vi "Process Init.vi"(0 "Process In":refnum<class "Process.lvclass">, 7 "Process Name":string, 11 "Error In":errorcluster) -> (4 "Process Out":refnum<class "Process.lvclass">, 15 "Error Out":errorcluster)   [LabVIEW 2023, in "Process.lvclass"]
doc: "Initializes new process by naming and starting it."
uses:
  Process.lvclass
  Process.lvclass/Process.ctl
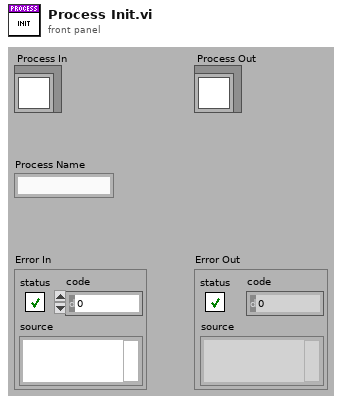
[diagram p1: front panel]
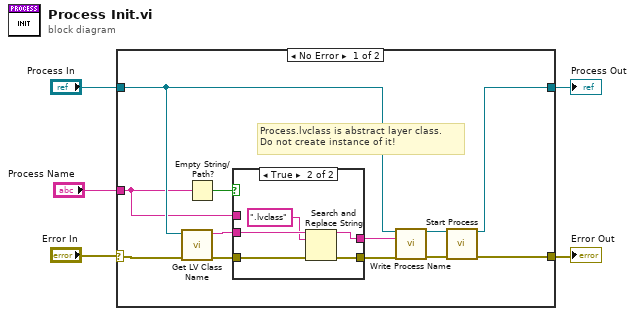
[diagram p0: block diagram]
diagram:
  n1 = case shown="No Error" "Error In" {
    selector: "Error In" -> [w10 w25]
    tunnel: "Process In" -> [w13 w26]
    tunnel: [w16 w26] -> w4
    tunnel: [w17 w25] -> w2
    tunnel: "Process Name" -> [w6 _]
    frame No Error {
      # "Process.lvclass is abstract layer class. \nDo not create instance of it!"
      n2 = call <vilib>:"Get LV Class Name.vi"("error in (no error)"=w10, "object"=w13) -> ("error out"=w9:errorcluster, "class name"=w11:string)  [unwired: 8 in]
      n3 = Empty String/Path?(string/path=w6) -> (empty?=w7:bool)
      n4 = case shown="True" w7 {
        tunnel: w6 -> [w19 _]
        tunnel: [w19 w22] -> w12
        tunnel: w11 -> [_ w24]
        tunnel: w9 -> [w18 w21]
        tunnel: [w18 w20] -> w8
        frame False {
        }
        frame True {
          n5 = Search and Replace String(input string=w24, search string=".lvclass", error in=w21) -> (result string=w22:string, error out=w20:errorcluster)  [unwired: 5 in, 2 out]
        }
      }
      n6 = call "Write Process Name.vi"("Process Out"=w13, "Process Name"=w12, "Error In"=w8) -> ("Process Out"=w15:refnum<class "Process.lvclass">, "Error Out"=w14:errorcluster)  [unwired: 11 in]
      n7 = call-dynamic "Start Process.vi"("Process In"=w15, "Error In"=w14) -> ("Process Out"=w16:refnum<class "Process.lvclass">, "Error In"=w17:errorcluster)  [unwired: 11 in, 1 out]
    }
    frame Error {
    }
  }
  "Process Out" <- w4
  "Error Out" <- w2
